vi "Global 213.vi"() -> ()   [LabVIEW 2013]
panel:
  out "Beam ON":bool
  in  "NMR Channel":i32=3 min=0 max=7 step=1
  in  "TEQ Comment":string="Unused"
  in  "Q Comment":string="Unused"
  in  "TEQ file":string="NMRave.xls"
  in  "Measurement":enum16{"TEQ", "POL", "QCV"}(ring)
  in  "Commentary":string="213 MHz crystal, SMT03 RF Gen"
  in  "Calib Constant":dbl=1.0 min=0.0 max=1.0 step=0.001 format="%_3f"
  out "File name":string="C:\\users\\plm\\Desktop\\rssmt\\data\\TEQ3559320656.csv"
  in  "IP Address":string="192.168.0.4"
  in  "Gain":enum16{"LOW", "HI", "MAX"}(ring)=enum."MAX"
  in  "COM Port #":refnum<visa-resource-name>="COM8"
  out "Peak center (MHz)":sgl=212.7195 format="%.3f"
  in  "Logoffset (V)":dbl=-5.38 min=-9.0 max=0.0 step=0.0005 format="%_5g"
  in  "Phase (V)":dbl=4.80000000000001 min=0.0 max=10.7 step=0.0005 format="%_5g"
  in  "Real/Quad Q curve":bool=TRUE
  out "Temperature (C)":dbl(graph)=25.25
  out "+3V supply":dbl=3.279 format="%_4g"
  out "Temp (C)":dbl=25.25 format="%_4g"
  in  "RemovePed":bool=TRUE
  in  "IF / LOG Det":bool
  in  "Q curve file":string="NMRave.xls"
  in  "AutoTune":bool=TRUE
  out "RF OK":bool=TRUE
  out "Peak area (mV-MHz)":sgl=0.38502613 format="%.5f"
  in  "Gauss Fit":bool
  out "NMR Graph + Fit":cluster{cluster{dbl, "Numeric":dbl}[]}[](graph)=[{[{212.6, "Numeric"=-0.015303813333331551}, {212.60399999999998, "Numeric"=-0.013759813333332833}, {212.608, "Numeric"=-0.013221253333330282}, {212.612, "Numeric"=-0.012688133333331547}, {212.61599999999999, "Numeric"=-0.013160453333332786}, {212.62, "Numeric"=-0.013638213333330313}, {212.624, "Numeric"=-0.013121413333331547}, {212.628, "Numeric"=-0.013610053333332747}, {212.632, "Numeric"=-0.013104133333330353}, {212.636, "Numeric"=-0.01160365333333155}, {212.64, "Numeric"=-0.012108613333332713}, {212.644, "Numeric"=-0.011619013333330395}, {212.648, "Numeric"=-0.011134853333331553}, {212.652, "Numeric"=-0.01165613333333268}, {212.656, "Numeric"=-0.011182853333330443}, {212.66, "Numeric"=-0.010715013333331563}, {212.664, "Numeric"=-0.011252613333332653}, {212.668, "Numeric"=-0.010795653333330492}, {212.672, "Numeric"=-0.009344133333331572}, {212.676, "Numeric"=-0.007898053333332631}, {212.68, "Numeric"=-0.007457413333330546}, {212.684, "Numeric"=-0.006022213333331587}, {212.688, "Numeric"=-0.0035924533333326096}, {212.692, "Numeric"=-0.0011681333333306003}, {212.696, "Numeric"=0.002250746666668393}, {212.7, "Numeric"=0.007664186666667411}, {212.704, "Numeric"=0.014072186666669335}, {212.708, "Numeric"=0.022474746666668367}, {212.712, "Numeric"=0.03187186666666743}, {212.716, "Numeric"=0.04026354666666927}, {212.72, "Numeric"=0.04264978666666835}, {212.724, "Numeric"=0.038030586666667435}, {212.728, "Numeric"=0.029405946666666547}, {212.732, "Numeric"=0.01977586666666831}, {212.736, "Numeric"=0.012140346666667438}, {212.74, "Numeric"=0.006499386666666599}, {212.744, "Numeric"=0.0018529866666682725}, {212.748, "Numeric"=-0.0007988533333325558}, {212.752, "Numeric"=-0.0024561333333333627}, {212.756, "Numeric"=-0.003118853333331767}, {212.76, "Numeric"=-0.00278701333333256}, {212.764, "Numeric"=-0.0014606133333333268}, {212.768, "Numeric"=-0.00013965333333180768}, {212.772, "Numeric"=0.002175866666667436}, {212.776, "Numeric"=0.005485946666666707}, {212.78, "Numeric"=0.010790586666668147}, {212.784, "Numeric"=0.01708978666666743}, {212.788, "Numeric"=0.02538354666666674}, {212.792, "Numeric"=0.0326718666666681}, {212.796, "Numeric"=0.03595474666666742}, {212.79999999999998, "Numeric"=0.03423218666666676}, {212.804, "Numeric"=0.02850418666666804}, {212.808, "Numeric"=0.0207707466666674}, {212.81199999999998, "Numeric"=0.013031866666666782}, {212.816, "Numeric"=0.008287546666667985}, {212.82, "Numeric"=0.0045377866666673795}, {212.82399999999998, "Numeric"=0.0017825866666667989}, {212.828, "Numeric"=0.0010219466666679256}, {212.832, "Numeric"=0.0002558666666673561}, {212.83599999999998, "Numeric"=-0.0005156533333331864}, {212.84, "Numeric"=0.00270738666666786}, {212.844, "Numeric"=0.005924986666667329}, {212.84799999999998, "Numeric"=0.010137146666666822}, {212.852, "Numeric"=0.013343866666667792}, {212.856, "Numeric"=0.0155451466666673}, {212.85999999999999, "Numeric"=0.01374098666666683}, {212.864, "Numeric"=0.01093138666666772}, {212.868, "Numeric"=0.006116346666667264}, {212.87199999999999, "Numeric"=0.0012958666666668332}, {212.876, "Numeric"=-0.0015300533333323545}, {212.88, "Numeric"=-0.0033614133333327734}, {212.884, "Numeric"=-0.004198213333333168}, {212.888, "Numeric"=-0.005040453333332434}, {212.892, "Numeric"=-0.0038881333333328156}, {212.896, "Numeric"=-0.0027412533333331717}, {212.9, "Numeric"=-0.0005998133333325166}, {212.904, "Numeric"=0.001536186666667139}, {212.908, "Numeric"=0.004666746666666821}, {212.912, "Numeric"=0.007791866666667397}, {212.916, "Numeric"=0.008911546666667089}, {212.92, "Numeric"=0.008025786666666807}, {212.924, "Numeric"=0.007134586666667307}, {212.928, "Numeric"=0.005237946666667038}, {212.932, "Numeric"=0.0033358666666667936}, {212.936, "Numeric"=0.0024283466666672133}, {212.94, "Numeric"=-0.000484613333333019}, {212.944, "Numeric"=-0.0024030133333332255}, {212.948, "Numeric"=-0.003326853333332885}, {212.952, "Numeric"=-0.0032561333333330795}, {212.956, "Numeric"=-0.002190853333333248}, {212.96, "Numeric"=-0.00013101333333298613}, {212.964, "Numeric"=0.004923386666666857}, {212.968, "Numeric"=0.010972346666666724}, {212.972, "Numeric"=0.016015866666666906}, {212.976, "Numeric"=0.021053946666666788}, {212.98, "Numeric"=0.023086586666666697}, {212.984, "Numeric"=0.020113786666666626}, {212.988, "Numeric"=0.015135546666666718}, {212.992, "Numeric"=0.009151866666666661}, {212.996, "Numeric"=0.004162746666666631}, {213.0, "Numeric"=-0.0008318133333333564}, {213.004, "Numeric"=-0.0038318133333333755}, {213.008, "Numeric"=-0.005837253333333369}, {213.012, "Numeric"=-0.006848133333333435}, {213.016, "Numeric"=-0.007864453333333417}, {213.02, "Numeric"=-0.007886213333333374}, {213.024, "Numeric"=-0.006913413333333517}, {213.028, "Numeric"=-0.005946053333333461}, {213.032, "Numeric"=-0.003984133333333381}, {213.036, "Numeric"=-2.7653333333603003e-05}, {213.04, "Numeric"=0.00492338666666649}, {213.044, "Numeric"=0.008868986666666606}, {213.048, "Numeric"=0.010809146666666306}, {213.052, "Numeric"=0.009743866666666438}, {213.056, "Numeric"=0.006673146666666592}, {213.06, "Numeric"=0.001596986666666214}, {213.064, "Numeric"=-0.002484613333333618}, {213.068, "Numeric"=-0.005571653333333425}, {213.072, "Numeric"=-0.007664133333333883}, {213.076, "Numeric"=-0.007762053333333677}, {213.08, "Numeric"=-0.007865413333333448}, {213.084, "Numeric"=-0.005974213333333984}, {213.088, "Numeric"=-0.0040884533333337405}, {213.092, "Numeric"=-0.001208133333333473}, {213.096, "Numeric"=-0.0003332533333340877}, {213.1, "Numeric"=0.0005361866666661926}, {213.104, "Numeric"=0.00040018666666649725}, {213.108, "Numeric"=-0.0007412533333341958}, {213.112, "Numeric"=-0.002888133333333878}, {213.116, "Numeric"=-0.0050404533333335355}, {213.12, "Numeric"=-0.007198213333334307}, {213.124, "Numeric"=-0.008361413333333952}, {213.12800000000001, "Numeric"=-0.008530053333333572}, {213.132, "Numeric"=-0.009704133333334425}, {213.136, "Numeric"=-0.00888365333333403}, {213.14000000000001, "Numeric"=-0.008068613333333613}, {213.144, "Numeric"=-0.007259013333334541}, {213.148, "Numeric"=-0.005454853333334113}, {213.15200000000002, "Numeric"=-0.0026561333333336573}, {213.156, "Numeric"=0.00013714666666533501}, {213.16, "Numeric"=0.0019249866666658031}, {213.16400000000002, "Numeric"=0.0007073866666662957}, {213.168, "Numeric"=-0.000515653333334791}, {213.172, "Numeric"=-0.0007441333333342859}, {213.17600000000002, "Numeric"=2.1946666666243812e-05}, {213.18, "Numeric"=0.001782586666665078}, {213.184, "Numeric"=0.0055377866666656205}, {213.18800000000002, "Numeric"=0.008287546666666187}, {213.192, "Numeric"=0.011031866666664943}, {213.196, "Numeric"=0.010770746666665524}, {213.2, "Numeric"=0.008504186666666129}, {213.204, "Numeric"=0.006232186666664808}, {213.208, "Numeric"=0.003954746666665424}, {213.212, "Numeric"=0.002671866666666067}, {213.216, "Numeric"=0.00038354666666466706}, {213.22, "Numeric"=-0.0009102133333346804}, {213.224, "Numeric"=-0.0012094133333339998}, {213.228, "Numeric"=-0.000514053333333293}, {213.232, "Numeric"=-0.0008241333333347857}, {213.236, "Numeric"=-0.00013965333333406976}, {213.24, "Numeric"=0.0005393866666666732}, {213.244, "Numeric"=0.0012129866666651015}, {213.248, "Numeric"=0.0008811466666658562}, {213.252, "Numeric"=-0.0004561333333333629}, {213.256, "Numeric"=-0.001798853333335013}, {213.26, "Numeric"=-0.004147013333334222}, {213.264, "Numeric"=-0.006500613333333401}, {213.268, "Numeric"=-0.007859653333335131}, {213.272, "Numeric"=-0.008224133333334303}, {213.276, "Numeric"=-0.008594053333333448}, {213.28, "Numeric"=-0.007969413333335252}, {213.284, "Numeric"=-0.008350213333334385}, {213.288, "Numeric"=-0.008736453333333494}, {213.292, "Numeric"=-0.00812813333333538}, {213.296, "Numeric"=-0.007525253333334475}, {213.3, "Numeric"=-0.006927813333333545}, {213.304, "Numeric"=-0.007335813333335508}, {213.308, "Numeric"=-0.007749253333334567}, {213.312, "Numeric"=-0.0091681333333336}, {213.316, "Numeric"=-0.011592453333335643}, {213.32, "Numeric"=-0.013022213333334661}, {213.324, "Numeric"=-0.014457413333333658}, {213.328, "Numeric"=-0.014898053333335777}, {213.332, "Numeric"=-0.015344133333334762}, {213.336, "Numeric"=-0.014795653333333719}, {213.34, "Numeric"=-0.014252613333335922}, {213.344, "Numeric"=-0.012715013333334866}, {213.348, "Numeric"=-0.012182853333333786}, {213.352, "Numeric"=-0.009656133333336063}, {213.356, "Numeric"=-0.007134853333334973}, {213.36, "Numeric"=-0.003619013333333857}, {213.364, "Numeric"=-0.00110861333333621}, {213.368, "Numeric"=0.002396346666664919}, {213.372, "Numeric"=0.003895866666666075}, {213.376, "Numeric"=0.0033899466666636397}, {213.38, "Numeric"=-0.00012141333333519984}, {213.38400000000001, "Numeric"=-0.0036382133333340066}, {213.388, "Numeric"=-0.00816045333333652}, {213.392, "Numeric"=-0.011688133333335314}, {213.39600000000002, "Numeric"=-0.014221253333334084}, {213.4, "Numeric"=-0.01575981333333668}]}]
  in  "Amp of Q curve":dbl=0.1699999999999999 min=0.0 max=1000.0 step=0.01 format="%_3f"
  in  "Subtract Q curve":bool=TRUE
  out "Pedestal Offset":dbl(graph)=0.0018311333333333693
  out "Pedestal Difference":dbl(graph)=-0.008016480000002515
  out "# Good Spectra":i32=988
  in  "Quality cuts":bool=TRUE
  out "Pedestal OK":bool=TRUE
  out "Sweep #":i32=244
  out "1st Sweep":bool
  out "ADC volts OK":bool=TRUE
  out "Peak Height Distribution":cluster{"Y":dbl[], "Y":dbl[]}[](graph)=[{"Y"=[0.042160036666668343, 0.04219720333333501, 0.04223437000000167, 0.042271536666668344, 0.04230870333333501, 0.04234587000000167, 0.042383036666668344, 0.04242020333333501, 0.042457370000001673, 0.042494536666668345, 0.04253170333333501, 0.042568870000001674, 0.04260603666666834, 0.04264320333333501, 0.042680370000001674, 0.04271753666666834, 0.04275470333333501, 0.042791870000001675, 0.04282903666666834, 0.04286620333333501, 0.042903370000001675, 0.04294053666666834, 0.04297770333333501, 0.043014870000001676, 0.04305203666666834, 0.04308920333333501, 0.043126370000001676, 0.04316353666666834, 0.04320070333333501, 0.04323787000000168, 0.04327503666666834, 0.04331220333333501, 0.04334937000000168, 0.04338653666666834, 0.04342370333333501, 0.04346087000000168, 0.04349803666666834, 0.04353520333333501, 0.04357237000000168, 0.04360953666666834, 0.04364670333333501, 0.04368387000000168, 0.04372103666666834, 0.04375820333333501, 0.04379537000000168, 0.043832536666668344, 0.04386970333333501, 0.04390687000000168, 0.043944036666668344, 0.04398120333333501, 0.04401837000000168, 0.044055536666668345, 0.04409270333333501, 0.04412987000000168, 0.044167036666668345, 0.04420420333333501, 0.04424137000000168, 0.044278536666668346, 0.04431570333333501, 0.04435287000000168, 0.044390036666668346, 0.04442720333333501, 0.044464370000001675, 0.04450153666666835, 0.04453870333333501, 0.044575870000001676, 0.04461303666666835, 0.04465020333333501, 0.044687370000001676, 0.04472453666666835, 0.04476170333333501, 0.04479887000000168, 0.04483603666666835, 0.04487320333333501, 0.04491037000000168, 0.04494753666666835, 0.04498470333333501, 0.04502187000000168, 0.04505903666666835, 0.045096203333335014, 0.04513337000000168, 0.04517053666666835, 0.045207703333335014, 0.04524487000000168, 0.04528203666666835, 0.045319203333335015, 0.04535637000000168, 0.045393536666668344, 0.045430703333335015, 0.04546787000000168, 0.045505036666668344, 0.045542203333335016, 0.04557937000000168, 0.045616536666668345, 0.045653703333335016, 0.04569087000000168, 0.045728036666668345, 0.04576520333333502, 0.04580237000000168, 0.045839536666668346], "Y"=[1.0, 1.0, 2.0, 3.0, 2.0, 3.0, 3.0, 0.0, 5.0, 1.0, 3.0, 3.0, 2.0, 5.0, 2.0, 6.0, 5.0, 8.0, 4.0, 11.0, 8.0, 3.0, 10.0, 8.0, 12.0, 9.0, 13.0, 16.0, 18.0, 6.0, 12.0, 7.0, 12.0, 14.0, 22.0, 18.0, 12.0, 10.0, 17.0, 18.0, 19.0, 24.0, 19.0, 19.0, 18.0, 20.0, 20.0, 29.0, 14.0, 12.0, 14.0, 18.0, 23.0, 19.0, 19.0, 11.0, 19.0, 17.0, 16.0, 26.0, 25.0, 8.0, 12.0, 15.0, 8.0, 22.0, 19.0, 16.0, 8.0, 13.0, 16.0, 12.0, 11.0, 6.0, 7.0, 9.0, 12.0, 5.0, 10.0, 5.0, 7.0, 4.0, 5.0, 3.0, 5.0, 5.0, 4.0, 4.0, 1.0, 2.0, 2.0, 3.0, 1.0, 2.0, 3.0, 1.0, 2.0, 1.0, 2.0, 1.0]}]
  in  "# of Sweeps":i32=1000
  out "S/N":dbl=60.56893184534198 format="%_3g"
  out "Peak mean (V)":dbl=0.04397488788124324 format="%_4g"
  out "Peak Height":dbl(graph)=0.04264978666666835
  in  "Raw Data":bool=TRUE
  in  "Tank RF":bool=TRUE
  out "IF Atten (dB)":i8=10 min=0 max=31 step=1
  in  "IFoffset (V)":dbl=2.160090000000069 min=-0.0 max=9.0 step=0.001 format="%.4f"
  in  "Tune  (V)":dbl=0.5180000000000009 min=-0.5 max=8.0 step=0.001 format="%.4f"
  in  "Invert Polarity":bool=TRUE
  out "Pedestal Diff (V)":sgl=-0.00801648 format="%.3f"
  out "Peak amp (V)":sgl=0.042649787 format="%.4f"
  in  "Save Data to File":bool=TRUE
  out "RF Level (dBm)":dbl=9.0 min=-10.0 max=10.0 step=0.1 format="%.2f"
  out "Sample RMS (V)":dbl format="%.4f"
  in  "# Sample/step":i32=20 min=1 max=1000 step=1
  in  "Step Width (MHz)":dbl=0.004 min=0.0 max=1000.0 step=5e-05 format="%.5f"
  in  "Freq Span (MHz)":dbl=0.8 min=0.0 max=50.0 step=0.1 format="%.3f"
  in  "Center Freq (MHz)":dbl=213.0 min=150.0 max=250.0 step=0.1 format="%.3f"
  # "Settings"
  # "E1039 Global NMR Control Panel"
  # "R\nF\n\nG\nE\nN \n\n+\n\nI\nF"
  # "D\nA\nC\ns"
  # "A\nD\nC"
  # "I\n/\nO"
  # "D\nA\nT\nA\n\nA \nN\nA\nL\nY\nS\nI\nS"
  # "Polarization"
  # "/ Polarization %"
  # "Results"
  # "A\nv\ne\nr\na\ng\ne\ns"
  # "S\nw\ne\ne\np"
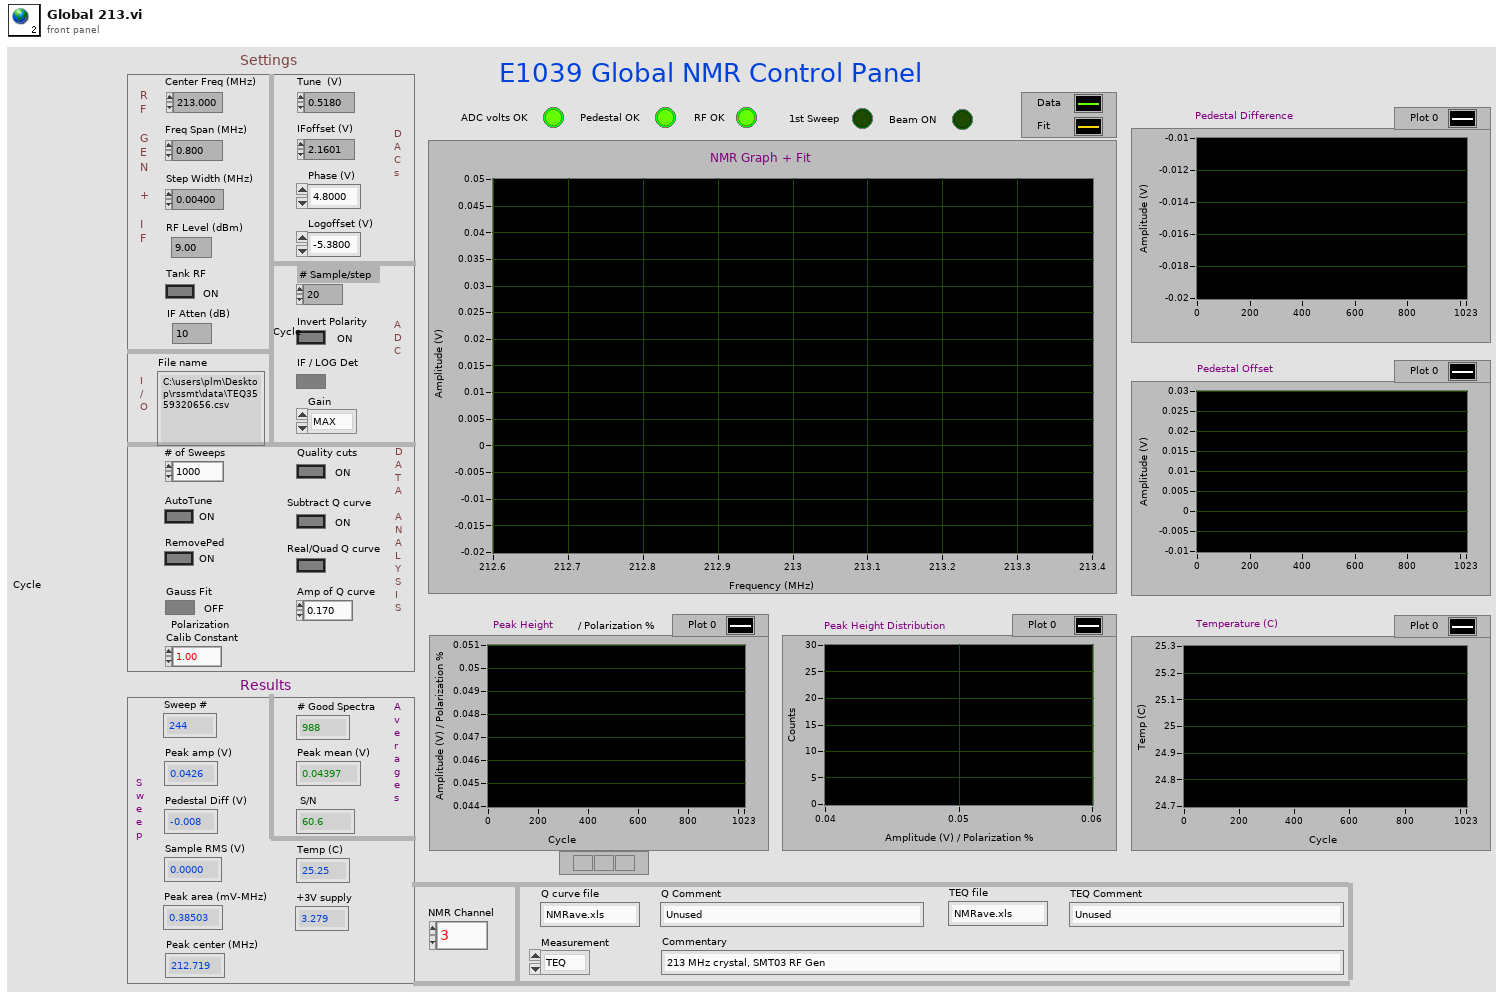
[diagram p1: front panel]
diagram:
